vi "ReadAcquiredSignals.vi"() -> ()   [LabVIEW 2025]
panel:
  out "signal characteristics":T1
  in  "y offset":dbl(slide)=0.001 min=-5.0 max=5.0 scale=-5.0..5.0
  in  "x axis size":dbl(slide)=107.429203539823 min=1e-05 max=10000000.0 scale=-1.0..4900.0
  in  "max y axis amplitude":dbl(slide)=5.0 min=1e-05 max=10.0 scale=0.0..10.0
  out "error out":errorcluster
  out "signal out":waveform(dbl)(graph)
  in  "error in":errorcluster
  in  "file path in":path
  in  "stop":bool
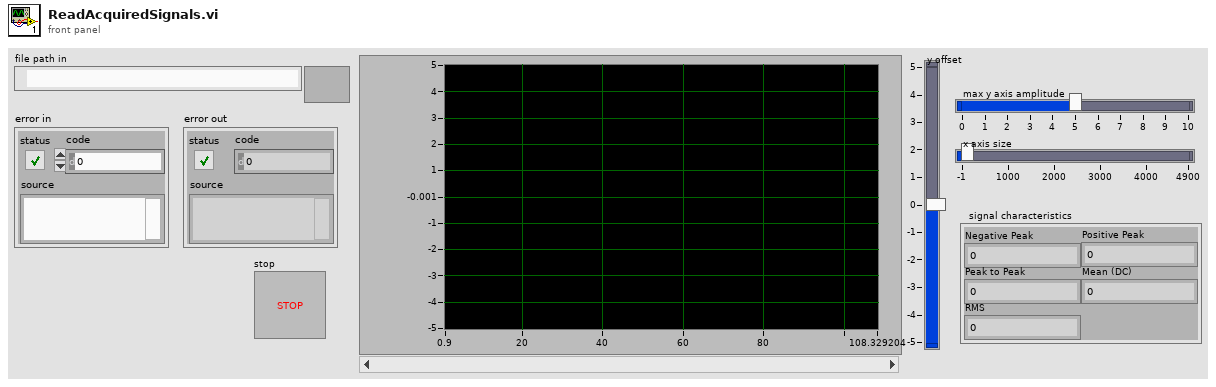
[diagram p1: front panel]
types:
  T1 = cluster{"Peak to Peak":dbl, "Positive Peak":dbl, "Negative Peak":dbl, "RMS":dbl, "Mean (DC)":dbl}
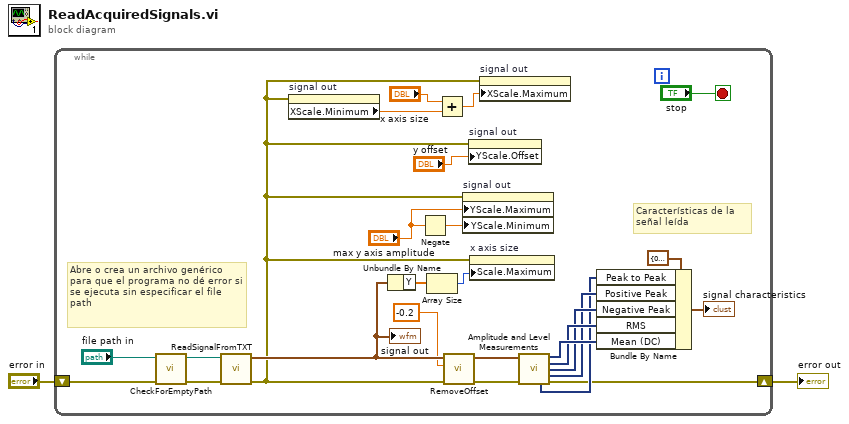
[diagram p0: block diagram]
diagram:
  n1 = while {
    shift-right: [w12] -> w2
    shift-left: "error in" -> [w4]
    stop <- "stop" stop-if-true
    # "Abre o crea un archivo genérico\npara que el programa no dé error si se ejecuta sin especificar el file path"
    # "Características de la señal leída"
    n2 = call "CheckForEmptyPath.vi"("error in (no error)"=w4, "file path in"="file path in") -> ("error out"=w6:errorcluster, "file path in"=w5:path)  [unwired: 8 in]
    n3 = call "ReadSignalFromTXT.vi"("error in"=w6, "file path in"=w5) -> ("error out"=w7:errorcluster, "signal out"=w10:waveform(dbl))  [unwired: 8 in]
    "signal out" <- w10
    n4 = property on="signal out" class="WFGraph (strict)"(error in=w7) -> ("XScale.Minimum"=w24:dbl)  [unwired: 1 in, 2 out]
    n5 = Unbundle By Name(w10) -> ("Y"=w21:dbl[])
    n6 = Negate(x="max y axis amplitude") -> (-x=w27:dbl)
    n7 = Array Size(array=w21) -> (size(s)=w22:i32)
    n8 = Add(x="x axis size", y=w24) -> (x+y=w23:dbl)
    n9 = call "RemoveOffset.vi"("error in"=w7, "offset value"=-0.2, "waveform"=w10) -> ("error out"=w11:errorcluster, "output waveform"=w9:waveform(dbl))  [unwired: 7 in]
    n10 = property on="signal out" class="WFGraph (strict)"(error in=w7, "YScale.Maximum"="max y axis amplitude", "YScale.Minimum"=w27) -> ()  [unwired: 1 in, 2 out]
    n11 = property on="signal out" class="WFGraph (strict)"(error in=w7, "YScale.Offset"="y offset") -> ()  [unwired: 1 in, 2 out]
    n12 = property on="x axis size" class="Slide (strict)"(error in=w7, "Scale.Maximum"=w22) -> ()  [unwired: 1 in, 2 out]
    n13 = property on="signal out" class="WFGraph (strict)"(error in=w7, "XScale.Maximum"=w23) -> ()  [unwired: 1 in, 2 out]
    n14 = call "Amplitude and Level Measurements"("Signals"=w9, "error in (no error)"=w11) -> ("Mean (DC)"=w17:dynamicdata, "RMS"=w16:dynamicdata, "Negative Peak"=w15:dynamicdata, "Positive Peak"=w14:dynamicdata, "Peak to Peak"=w13:dynamicdata, "error out"=w12:errorcluster)  [unwired: 8 in]
    n15 = Bundle By Name(cluster=T1 {"Peak to Peak"=0.0, "Positive Peak"=0.0, "Negative Peak"=0.0, "RMS"=0.0, "Mean (DC)"=0.0} ("signal properties"), "Peak to Peak"=w13, "Positive Peak"=w14, "Negative Peak"=w15, "RMS"=w16, "Mean (DC)"=w17) -> (→"signal characteristics":T1)
  }
  "error out" <- w2
